vi "DMM_Verify Instrument Options - Versions.vi"(8 "error in (no error)":errorcluster, 11 "3446X in":refnum<class "3446X.lvclass">) -> (0 "error out":errorcluster, 3 "3446X out":refnum<class "3446X.lvclass">)   [LabVIEW 2015, in "3446X.lvclass"]
uses:
  3446X.lvclass
  Controls/Instrument Attributes Cluster.ctl
  3446X.lvclass/3446X.ctl
  <instrlib>/Agilent 3446X Series/Agilent 3446X Series.lvlib
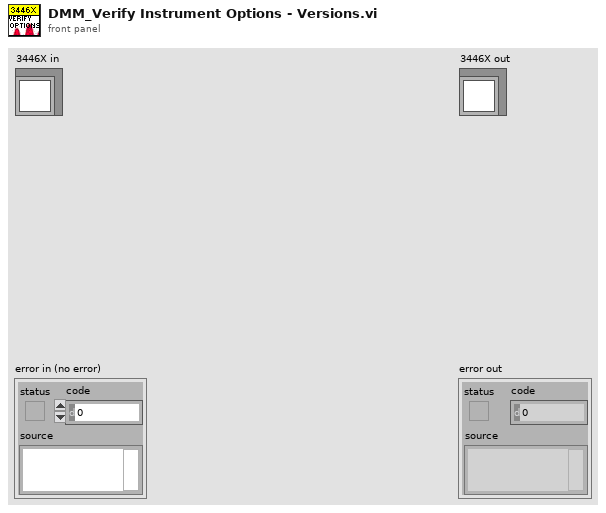
[diagram p1: front panel]
types:
  T1 = typedef "Instrument Attributes Cluster.ctl" = cluster{"Reported Firmware Rev":string, "Reported Options":string}
  T2 = typedef "Class Instrument Info.ctl" = string[]
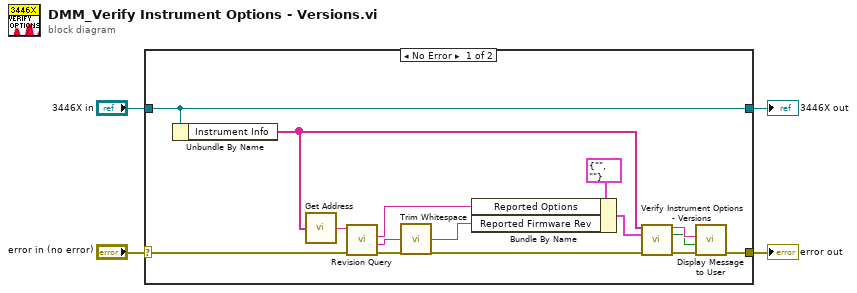
[diagram p0: block diagram]
diagram:
  n1 = case shown="No Error" "error in (no error)" {
    selector: "error in (no error)" -> [w10 w20]
    tunnel: [w15 w20] -> w4
    tunnel: [w14 w19] -> w1
    tunnel: "3446X in" -> [w14 w19]
    frame No Error {
      n2 = Unbundle By Name(w14) -> ("Instrument Info"=w5:T2)
      n3 = call "Get Address.vi"("Instrument Info"=w5) -> ("Address"=w6:string)  [unwired: 4 in]
      n4 = call <instrlib>:"Revision Query.vi"("error in (no error)"=w10, "VISA resource name"=w6) -> ("error out"=w9:errorcluster, "Instrument Firmware Revision"=w8:string, "Instrument Driver Revision"=w7:string)  [unwired: 6 in, 1 out]
      n5 = call <vilib>:"Trim Whitespace.vi"("string"=w8) -> ("trimmed string"=w12:string)  [unwired: 1 in]
      n6 = Bundle By Name(cluster=T1 {"Reported Firmware Rev"="", "Reported Options"=""} ("Instrument Attributes"), "Reported Options"=w7, "Reported Firmware Rev"=w12) -> (w11:T1)
      n7 = call "Verify Instrument Options - Versions.vi"("Instrument Info"=w5, "Instrument Attributes"=w11, "error in (no error)"=w9) -> ("Options & Versions Validation"=w18:string, "Mismatch? (True = Mismatch)"=w17:bool, "error out"=w16:errorcluster)  [unwired: 10 in]
      n8 = call "Display Message to User"("error in (no error)"=w16, "Enable"=w17, "Message"=w18) -> ("error out"=w15:errorcluster)  [unwired: 7 in, 1 out]
    }
    frame Error {
    }
  }
  "error out" <- w4
  "3446X out" <- w1
